vi "Read ADC.vi"(8 "error in (no error)":errorcluster, 10 "ADC Channel":dbl, 11 "object in":refnum<class "TI.lvclass">) -> (0 "error out":errorcluster, 3 "object out":refnum<class "TI.lvclass">)   [LabVIEW 2020, in "TI.lvclass"]
uses:
  TI.lvclass
  TI.lvclass/TI.ctl
  bda3f9ae-ebaa-4c7d-ac8b-a3eb4bd9c532.vi
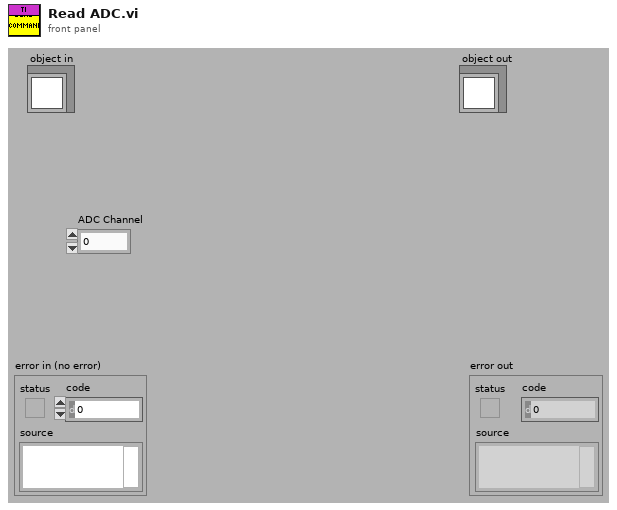
[diagram p1: front panel]
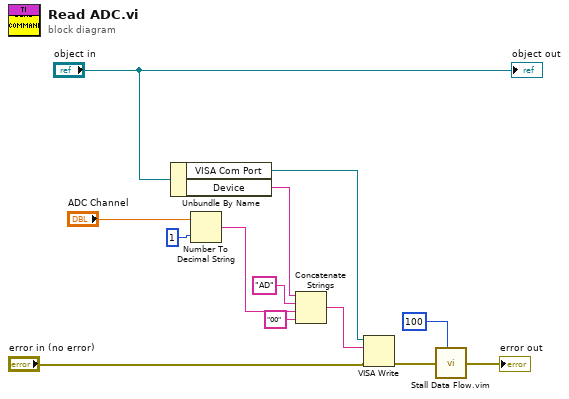
[diagram p0: block diagram]
diagram:
  n1 = Unbundle By Name("object in") -> ("VISA Com Port"=w12:refnum<visa-resource-name>, "Device"=w10:string)
  n2 = Number To Decimal String(number="ADC Channel", width (-)=i16 1) -> (decimal integer string=w9:string)
  n3 = Concatenate Strings(w10, "AD" ("string"), w9, "00" ("string")) -> (w11:string)
  n4 = VISA Write(VISA resource name=w12, write buffer=w11, error in (no error)="error in (no error)") -> (error out=w13:errorcluster)  [unwired: 2 out]
  n5 = call "Stall Data Flow.vim"("value in"=w13, "milliseconds to wait"=u32 100) -> ("value out"=→"error out":errorcluster)  [unwired: 1 out]
  "object out" <- "object in"
